vi "Handle and Broadcast Event.vi"(8 "error in (no error)":errorcluster, 9 "Event Data":refnum<class "Event.lvclass">, 10 "View Enqueuer":refnum<class "Message Enqueuer.lvclass">, 11 "Controller Actor in":refnum<class "Controller Actor.lvclass">) -> (0 "error out":errorcluster, 3 "Controller Actor out":refnum<class "Controller Actor.lvclass">)   [LabVIEW 2016, in "Event Actors.lvlib" / "Controller Actor.lvclass"]
doc: "This method generates/fires the Event wired to the input triggered by a View Actor. Firing an event originating form a View Actor looks up all actors, but the originating View, who Registered to listen to this Event and sends to them this Event on a Zero Coupling based message defined during Registration. Errors on broadcasting the event i.e. enqueuer of the registrant not existing, are ignored.\n\n<b>IMPORTANT</b> - Only call this method within the actor core of your Controller Actor. From helper loops call the Send Generate Event message to self. This is to make sure your actor works with all registered listeners."
uses:
  Controller Actor.lvclass
  <vilib>/ActorFramework/Message Enqueuer/Message Enqueuer.lvclass
  Event/Event.lvclass
  Controller Actor.lvclass/Controller Actor.ctl
  Event Handler Details.ctl
  Event Handlers/Event Generated Msg/Event Generated Msg.lvclass
  C:/Program Files (x86)/National Instruments/LabVIEW 2016/vi.lib/ActorFramework/Message/Message.lvclass
  Event Handlers/Event Generated Msg/Event Generated Msg.lvclass/Event Generated Msg.ctl
  <vilib>/ActorFramework/Message Enqueuer/Message Enqueuer.lvclass/Message Enqueuer.ctl
  <vilib>/ActorFramework/Message Enqueuer/Enqueue.vi
  <vilib>/Utility/LVClass/Get LV Class Name.vi
  <resource>/AFDebug/Generate Trace for Message.vi
  <vilib>/ActorFramework/Message Priority Queue/Priority Enqueue.vi
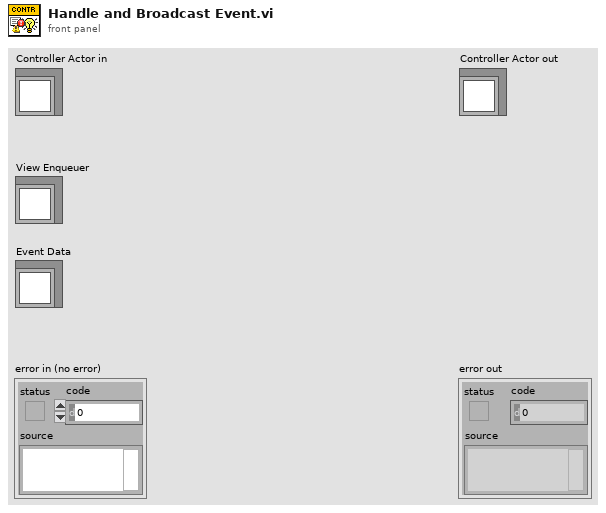
[diagram p1: front panel]
types:
  T1 = typedef "Event Actors.lvlib/Controller Actor.lvclass/Event Handler Details.ctl" = cluster{"Exclude From Broadcast":bool, "Paused":bool, "View Event Fire Handler":refnum<class "Event Generated Msg.lvclass">}
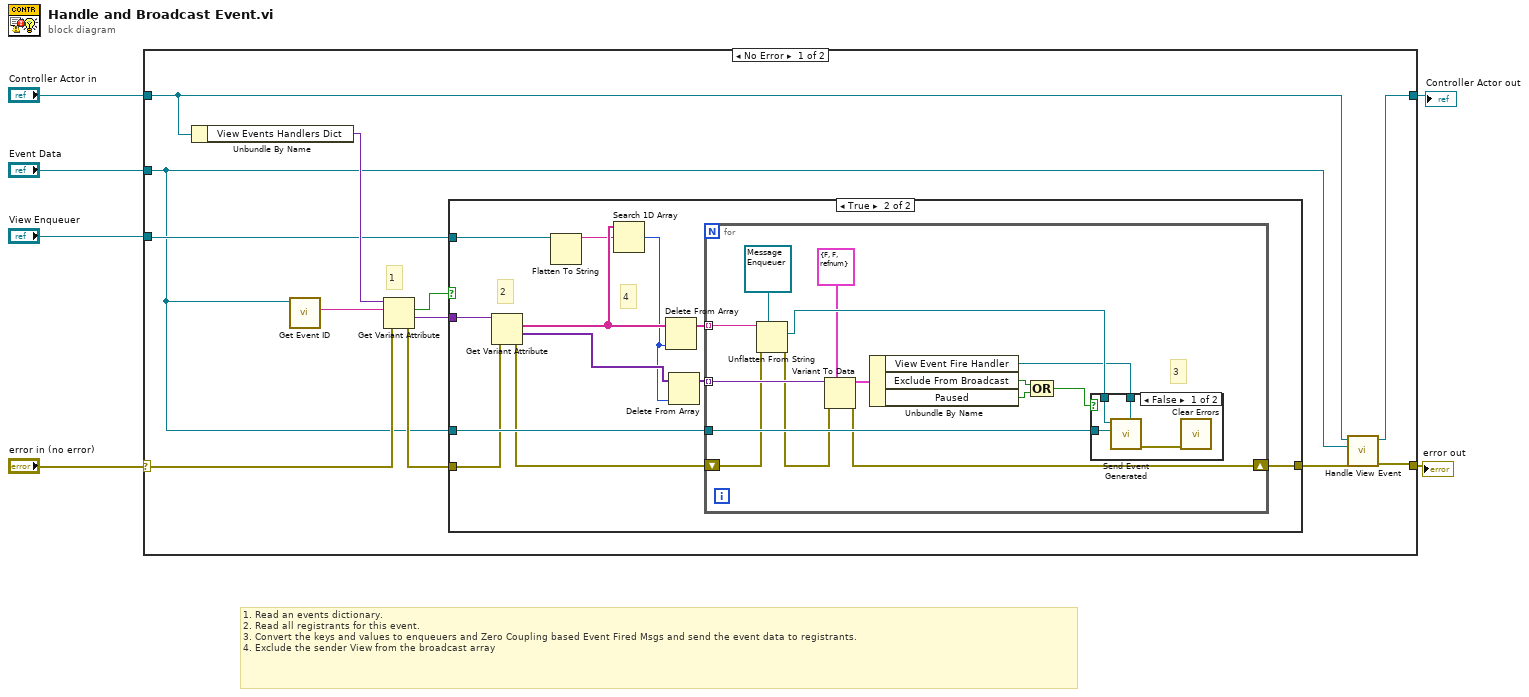
[diagram p0: block diagram]
diagram:
  # "1. Read an events dictionary.\n2. Read all registrants for this event.\n3. Convert the keys and values to enqueuers and Zero Coupling based Event Fired Msgs and send the event data to registrants.\n4. Exclude the sender View from the broadcast array"
  n1 = case shown="No Error" "error in (no error)" {
    selector: "error in (no error)" -> [w13 w51]
    tunnel: "Controller Actor in" -> [w9 w50]
    tunnel: "Event Data" -> [w7 _]
    tunnel: [w10 w51] -> w2
    tunnel: "View Enqueuer" -> [w12 _]
    tunnel: [w8 w50] -> w1
    frame No Error {
      # "1"
      n2 = Unbundle By Name(w9) -> ("View Events Handlers Dict"=w18:variant)
      n3 = call-dynamic "Get Event ID.vi"("Event in"=w7) -> ("Event ID"=w14:string)  [unwired: 8 in, 2 out]
      n4 = Get Variant Attribute(Variant=w18, name=w14, error in=w13) -> (found=w15:bool, value=w16:variant, error out=w17:errorcluster)  [unwired: 1 in, 1 out]
      n5 = case shown="True" w15 {
        tunnel: w16 -> [_ w29]
        tunnel: w7 -> [_ w31]
        tunnel: w17 -> [w19 w28]
        tunnel: [w19 w30] -> w11
        tunnel: w12 -> [_ w24]
        frame False {
        }
        frame True {
          # "4"
          # "2"
          n6 = Get Variant Attribute(Variant=w29, error in=w28) -> (names=w26:string[], values=w22:variant[], error out=w27:errorcluster)  [unwired: 2 in, 1 out]
          n7 = Flatten To String(anything=w24) -> (data string=w23:string)  [unwired: 3 in, 2 out]
          n8 = Search 1D Array(1D array=w26, element=w23) -> (index of element=w20:i32)  [unwired: 1 in]
          n9 = Delete From Array(array=w26, index=w20) -> (array with subset deleted=w25:string[])  [unwired: 1 in, 1 out]
          n10 = Delete From Array(array=w22, index=w20) -> (array with subset deleted=w21:variant[])  [unwired: 1 in, 1 out]
          n11 = for {
            tunnel: w25 -> [w45] mode=indexing
            tunnel: w21 -> [w44] mode=indexing
            tunnel: w31 -> [w41]
            shift-right: [w36] -> w30
            shift-left: w27 -> [w40]
            # "3"
            n12 = Unflatten From String(type=refnum<class "Message Enqueuer.lvclass"> refnum ("Message Enqueuer"), binary string=w45, error in (no error)=w40) -> (value=w43:refnum<class "Message Enqueuer.lvclass">, error out=w39:errorcluster)  [unwired: 2 in, 1 out]
            n13 = Variant To Data(error in=w39, type=T1 {"Exclude From Broadcast"=FALSE, "Paused"=FALSE, "View Event Fire Handler"=refnum} ("Message Type"), Variant=w44) -> (data=w42:T1, error out=w36:errorcluster)
            n14 = Unbundle By Name(w42) -> ("View Event Fire Handler"=w34:refnum<class "Event Generated Msg.lvclass">, "Exclude From Broadcast"=w33:bool, "Paused"=w32:bool)
            n15 = Compound Arithmetic op=OR(w33, w32) -> (w35:bool)
            n16 = case shown="False" w35 {
              tunnel: w34 -> [w49 _]
              tunnel: w41 -> [w48 _]
              tunnel: w43 -> [w46 _]
              frame False {
                n17 = call "Send Event Generated.vi"("Message Type"=w49, "Event Data"=w48, "Message Enqueuer"=w46) -> ("Error Out"=w47:errorcluster)  [unwired: 7 in, 1 out]
                n18 = call <vilib>:"Clear Errors.vi"("error in (no error)"=w47) -> ()  [unwired: 5 in, 2 out]
              }
              frame True {
              }
            }
          }
        }
      }
      n19 = call "Handle View Event.vi"("error in (no error)"=w11, "Event Data"=w7, "Controller Actor in"=w9) -> ("error out"=w10:errorcluster, "Controller Actor out"=w8:refnum<class "Controller Actor.lvclass">)  [unwired: 7 in]
    }
    frame Error {
    }
  }
  "error out" <- w2
  "Controller Actor out" <- w1
